vi "Save_Data.vi"(0 "保存路径":path=path "C:/Qmz/data1.bin", 3 "Save Data":bool) -> ()   [LabVIEW 2020]
uses:
  <vilib>/Platform/TimedLoop/XDataNode/timing_clust.ctl
  <vilib>/Platform/TimedLoop/XDataNode/nitl_modes.ctl
  <vilib>/Platform/TimedLoop/XDataNode/wakeup.ctl
  <vilib>/Platform/TimedLoop/XDataNode/XDataNode.xnode
  <vilib>/Platform/TimedLoop/XDataNode/XDNodeRunTimeDep.lvlib
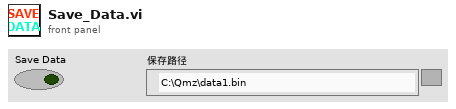
[diagram p1: front panel]
types:
  T1 = enum16{"open", "replace", "create", "open or create", "replace or create", "replace or create with confirmation"}
  T2 = typedef "XDNodeRunTimeDep.lvlib/timing_clust.ctl" = cluster{"Expected End [f-1]":u64, "Actual End [f-1]":u64, "Finished Late? [f-1]":bool, "Expected End [i-1]":u64, "Actual End [i-1]":u64, "Finished Late? [i-1]":bool, "Expected Start [i]":u64, "Actual Start [i]":u64, "Expected Start [f]":u64, "Actual Start [f]":u64, "Source Name":string, "Structure Name":string, "Period":i64, "Deadline":i64, "Offset":i64, "Start":i64, "Priority":i32, "Timeout":i32, "Mode":T3, "Wakeup Reason":T4, "Error":errorcluster, "Source Type":string, "Secondary Source Type":string, "Global End Time":u64, "Global Start Time":u64, "Frame Duration":u64, "Iteration Duration":u64, "Assigned CPU":i32, "I/O Scan Engine Mode":u32}
  T3 = typedef "XDNodeRunTimeDep.lvlib/nitl_modes.ctl" = enum32{"No Change", "Process missed periods, maintain original phase", "Discard missed periods, maintain original phase", "Process missed periods, ignore original phase", "Discard missed periods, ignore original phase"}
  T4 = typedef "XDNodeRunTimeDep.lvlib/wakeup.ctl" = enum32{"Normal", "Aborted", "Asynchronous wakeup", "Timing source error", "Timed loop error", "Timeout"}
  T5 = enum16{"big-endian, network order", "native, host order", "little-endian"}
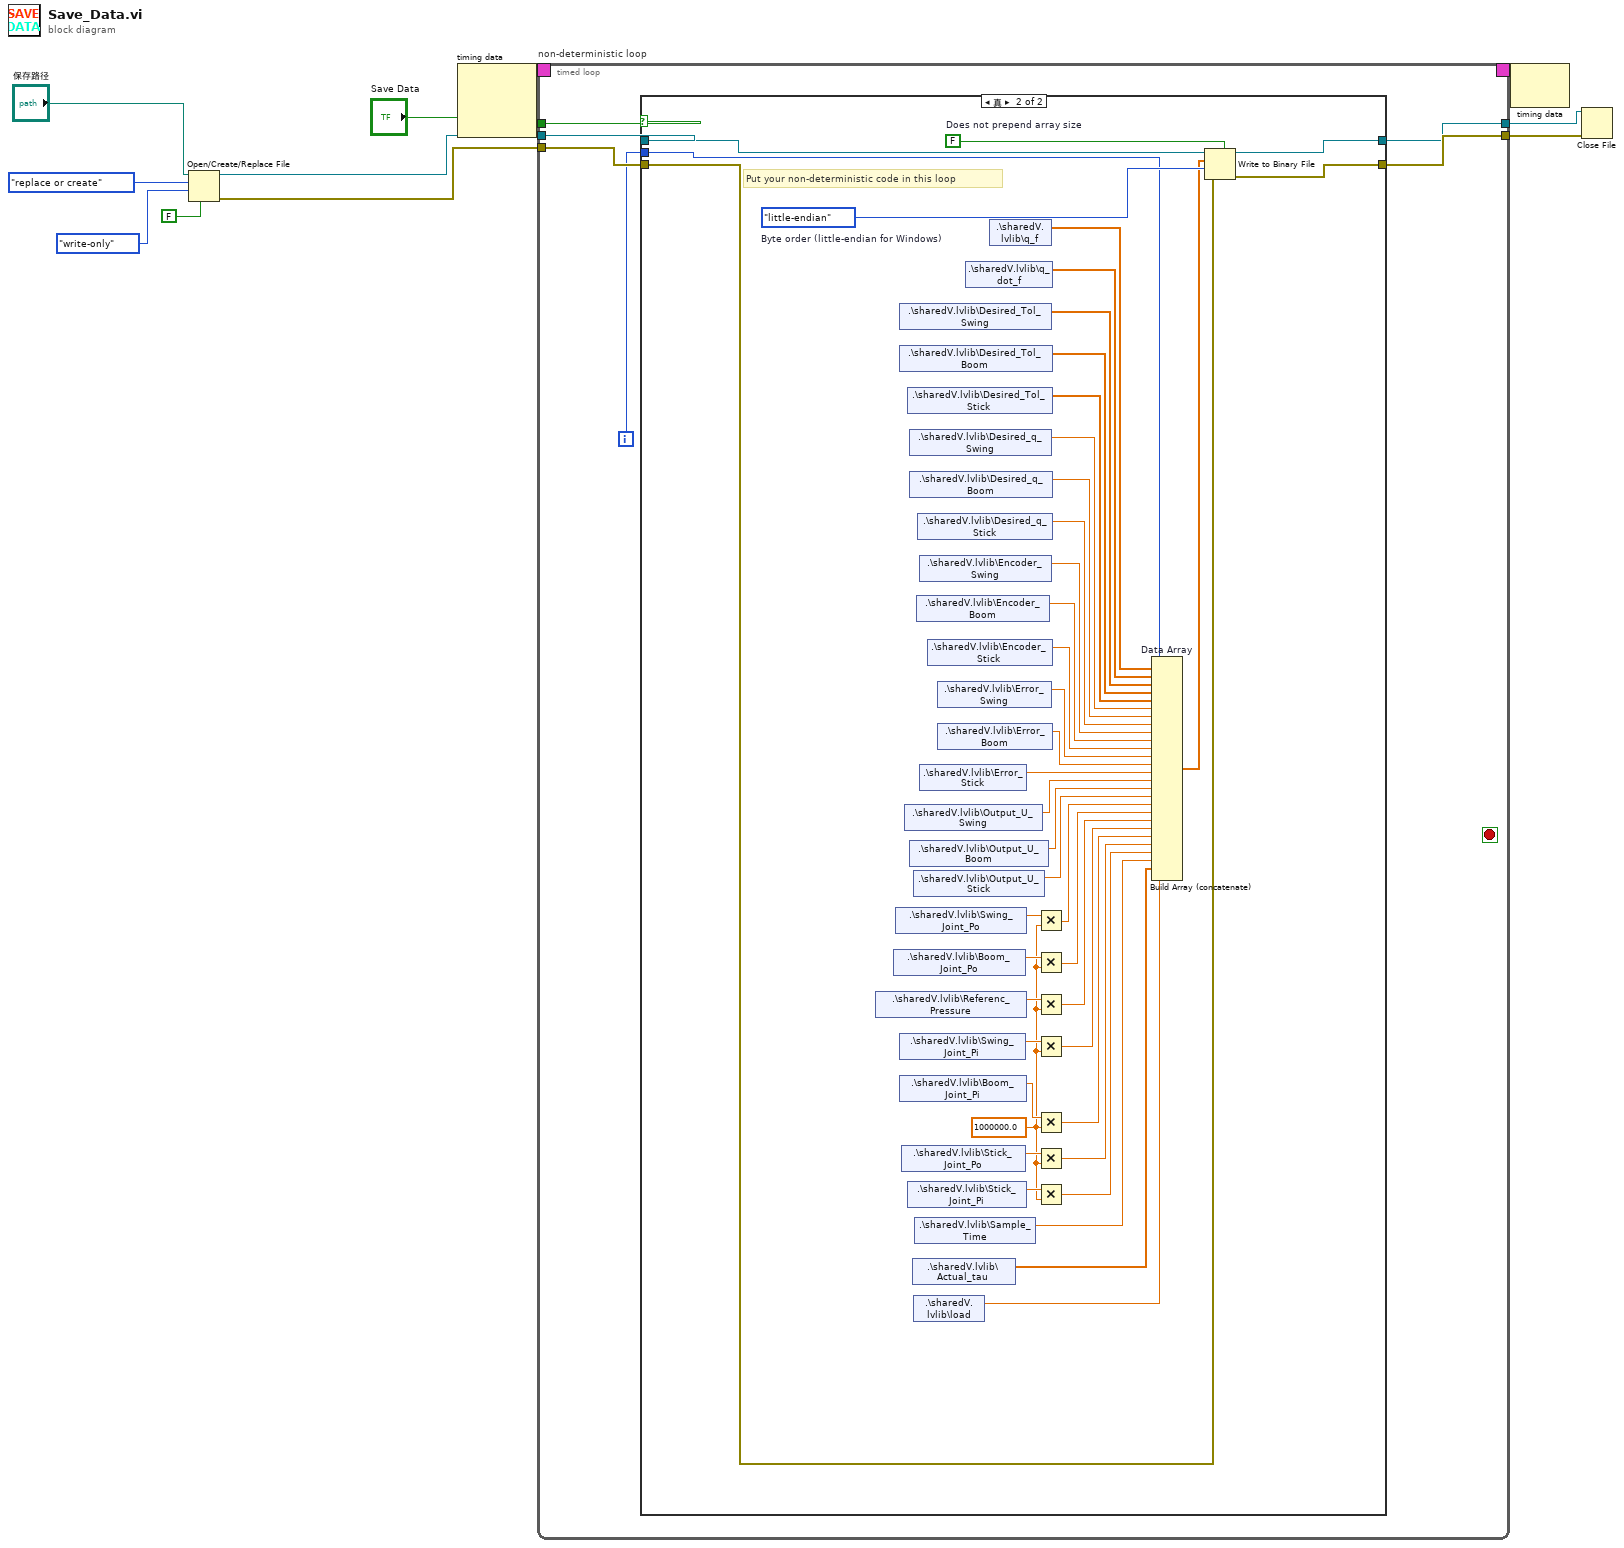
[diagram p0: block diagram]
diagram:
  n1 = Open/Create/Replace File(file path (use dialog)="保存路径", operation (0:open)=T1."replace or create", access (0:read/write)=enum16{"read/write", "read-only", "write-only"}."write-only" ("权限(0:read/write)"), disable buffering (F)=FALSE) -> (refnum out=w7:refnum<file>, error out=w6:errorcluster)  [unwired: 2 in, 1 out]
  n2 = node-c288 ("Input Node")() -> (w11:T2)  [unwired: 3 in]
  n3 = timed-loop "non-deterministic loop" {
    timing: w11 -> [_]
    timing-out: [_] -> w10
    tunnel: [w17] -> w4
    tunnel: w6 -> [w16]
    tunnel: [w15] -> w5
    tunnel: "Save Data" -> [w14]
    tunnel: w7 -> [w13]
    i -> [w12]
    stop <- _ stop-if-true
    n4 = case shown="真" w14 {
      tunnel: [w18 w62] -> w17
      tunnel: w13 -> [w19 w61]
      tunnel: w16 -> [w18 w60]
      tunnel: [w19 w57] -> w15
      tunnel: w12 -> [_ w55]
      frame False {
      }
      frame True {
        w33 = 1000000.0
        w58 = FALSE  # Does not prepend array size
        w59 = T5."little-endian"  # Byte order (little-endian for Windows)
        # "Put your non-deterministic code in this loop"
        n5 = shared-variable ".\\sharedV.lvlib\\Referenc_Pressure"() -> (w34:dbl)  [unwired: 1 in, 1 out]
        n6 = shared-variable ".\\sharedV.lvlib\\Boom_Joint_Po"() -> (w38:dbl)  [unwired: 1 in, 1 out]
        n7 = shared-variable ".\\sharedV.lvlib\\Swing_Joint_Po"() -> (w40:dbl)  [unwired: 1 in, 1 out]
        n8 = shared-variable ".\\sharedV.lvlib\\Desired_Tol_Swing"() -> (w52:dbl[])  [unwired: 1 in, 1 out]
        n9 = shared-variable ".\\sharedV.lvlib\\Desired_Tol_Boom"() -> (w51:dbl[])  [unwired: 1 in, 1 out]
        n10 = shared-variable ".\\sharedV.lvlib\\Swing_Joint_Pi"() -> (w39:dbl)  [unwired: 1 in, 1 out]
        n11 = shared-variable ".\\sharedV.lvlib\\Boom_Joint_Pi"() -> (w37:dbl)  [unwired: 1 in, 1 out]
        n12 = shared-variable ".\\sharedV.lvlib\\Stick_Joint_Po"() -> (w36:dbl)  [unwired: 1 in, 1 out]
        n13 = shared-variable ".\\sharedV.lvlib\\Output_U_Swing"() -> (w32:dbl)  [unwired: 1 in, 1 out]
        n14 = shared-variable ".\\sharedV.lvlib\\Desired_Tol_Stick"() -> (w50:dbl[])  [unwired: 1 in, 1 out]
        n15 = shared-variable ".\\sharedV.lvlib\\Stick_Joint_Pi"() -> (w35:dbl)  [unwired: 1 in, 1 out]
        n16 = shared-variable ".\\sharedV.lvlib\\Desired_q_Swing"() -> (w49:dbl)  [unwired: 1 in, 1 out]
        n17 = shared-variable ".\\sharedV.lvlib\\Desired_q_Boom"() -> (w48:dbl)  [unwired: 1 in, 1 out]
        n18 = shared-variable ".\\sharedV.lvlib\\Output_U_Boom"() -> (w31:dbl)  [unwired: 1 in, 1 out]
        n19 = shared-variable ".\\sharedV.lvlib\\Actual_tau"() -> (w21:dbl[])  [unwired: 1 in, 1 out]
        n20 = shared-variable ".\\sharedV.lvlib\\Output_U_Stick"() -> (w30:dbl)  [unwired: 1 in, 1 out]
        n21 = shared-variable ".\\sharedV.lvlib\\load"() -> (w20:dbl)  [unwired: 1 in, 1 out]
        n22 = shared-variable ".\\sharedV.lvlib\\Sample_Time"() -> (w22:dbl)  [unwired: 1 in, 1 out]
        n23 = shared-variable ".\\sharedV.lvlib\\Encoder_Boom"() -> (w45:dbl)  [unwired: 1 in, 1 out]
        n24 = shared-variable ".\\sharedV.lvlib\\Desired_q_Stick"() -> (w47:dbl)  [unwired: 1 in, 1 out]
        n25 = shared-variable ".\\sharedV.lvlib\\Encoder_Swing"() -> (w46:dbl)  [unwired: 1 in, 1 out]
        n26 = shared-variable ".\\sharedV.lvlib\\Error_Stick"() -> (w41:dbl)  [unwired: 1 in, 1 out]
        n27 = shared-variable ".\\sharedV.lvlib\\Encoder_Stick"() -> (w44:dbl)  [unwired: 1 in, 1 out]
        n28 = shared-variable ".\\sharedV.lvlib\\Error_Swing"() -> (w43:dbl)  [unwired: 1 in, 1 out]
        n29 = shared-variable ".\\sharedV.lvlib\\Error_Boom"() -> (w42:dbl)  [unwired: 1 in, 1 out]
        n30 = shared-variable ".\\sharedV.lvlib\\q_dot_f"() -> (w53:dbl[])  [unwired: 1 in, 1 out]
        n31 = shared-variable ".\\sharedV.lvlib\\q_f"() -> (w54:dbl[])  [unwired: 1 in, 1 out]
        n32 = Multiply(x=w40, y=w33) -> (x*y=w29:dbl)
        n33 = Multiply(x=w38, y=w33) -> (x*y=w28:dbl)
        n34 = Multiply(x=w34, y=w33) -> (x*y=w27:dbl)
        n35 = Multiply(x=w39, y=w33) -> (x*y=w26:dbl)
        n36 = Multiply(x=w37, y=w33) -> (x*y=w25:dbl)
        n37 = Multiply(x=w36, y=w33) -> (x*y=w24:dbl)
        n38 = Multiply(x=w35, y=w33) -> (x*y=w23:dbl)
        n39 = Build Array (concatenate) "Data Array"(w55, w54, w53, w52, w51, w50, w49, w48, w47, w46, w45, w44, w43, w42, w41, w32, w31, w30, w29, w28, w27, w26, w25, w24, w23, w22, w21, w20) -> (w56:dbl[])
        n40 = Write to Binary File(file (use dialog)=w61, data=w56, error in=w60, 5:w58, 9:w59) -> (refnum out=w57:refnum<file>, error out=w62:errorcluster)  [unwired: 1 in, 1 out]
      }
    }
  }
  n41 = node-c288 ("Output Node")(w10) -> ()  [unwired: 1 out]
  n42 = Close File(refnum=w5, error in=w4) -> ()  [unwired: 2 out]
